vi "AirQualityViewer.vi"() -> ()   [LabVIEW 2020]
uses:
  Ctrls/StateMachineEnum.ctl
  Ctrls/ProgData.ctl
  user32.dll
panel:
  in  "Reload":bool
  in  "Settings":bool
  in  "Close":bool
  out "TitleBar":bool
  out "Data":timestamp format="%<%H:%M %d/%m/%y>T"
  out "Value":dbl
  out "Main Graph":cluster{timestamp[], dbl[]}[](graph)
  in  "Sensors":u16(ring) items=["dwutlenek azotu", "ozon"]
  # "Mierzony parametr:"
  # "Zaznaczony punkt:"
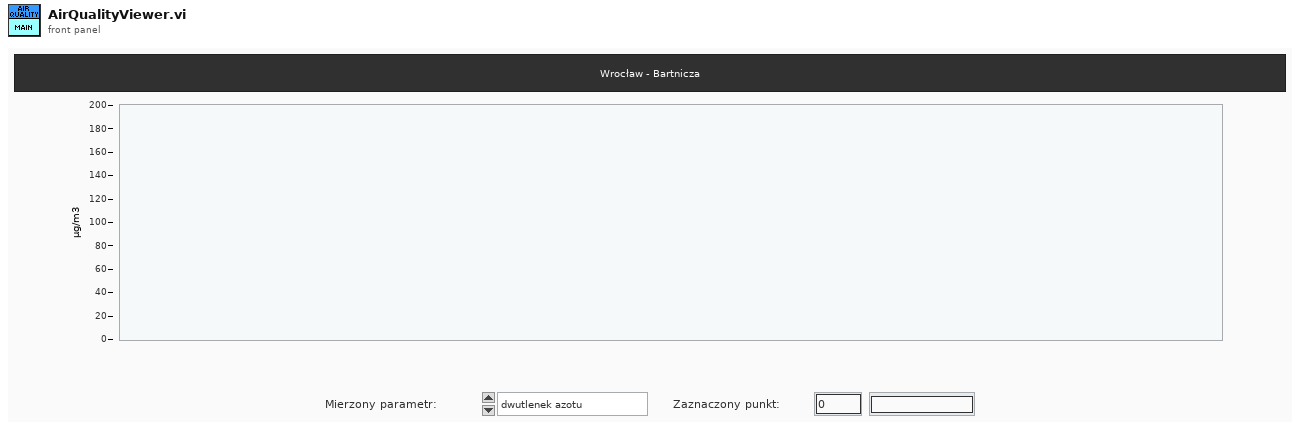
[diagram p1: front panel]
types:
  T1 = typedef "ProgData.ctl" = cluster{"Station":string[], "Sensor List":string[], "Sensor Id":dbl[], "Parameters":string[], "Values":i32[]}
  T2 = typedef "StateMachineEnum.ctl" = enum16{"INIT", "IDLE", "GET DATA", "ERROR HANDLER", "CLOSE"}
  T3 = typedef "LVPointDoubleTypeDef.ctl" = cluster{"Cursor X":dbl, "Cursor Y":dbl}
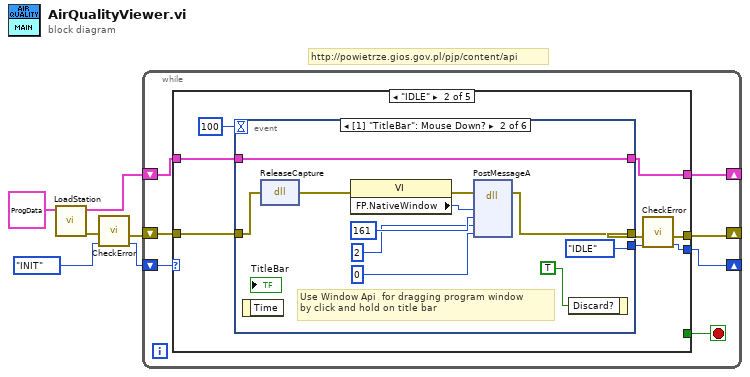
[diagram p0: block diagram]
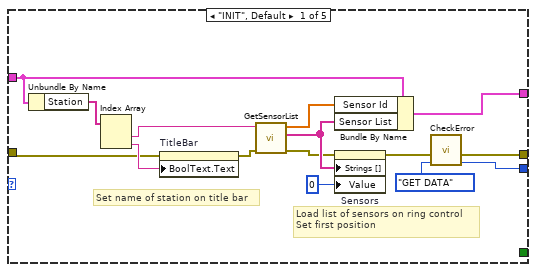
[diagram p2: hidden frame]
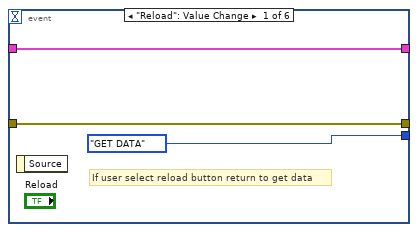
[diagram p3: hidden frame]
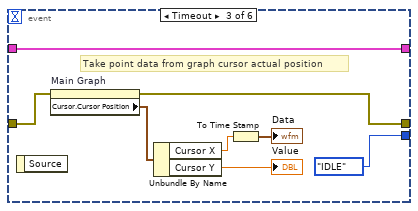
[diagram p4: hidden frame]
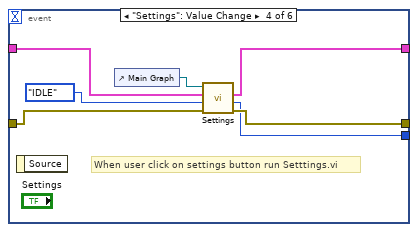
[diagram p5: hidden frame]
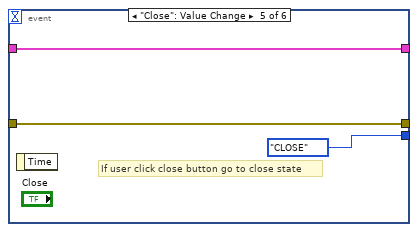
[diagram p6: hidden frame]
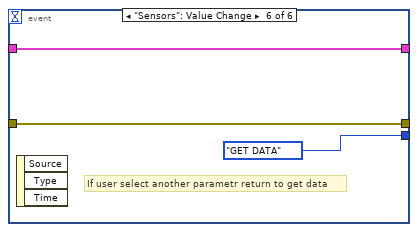
[diagram p7: hidden frame]
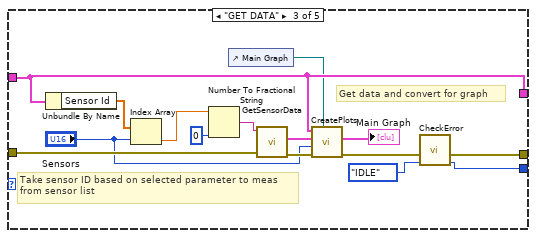
[diagram p8: hidden frame]
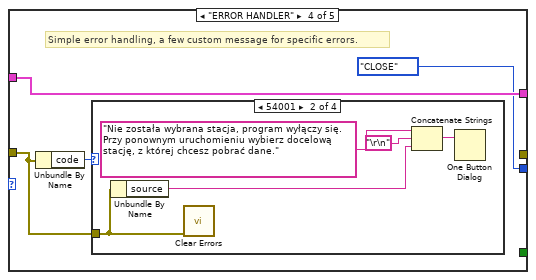
[diagram p9: hidden frame]
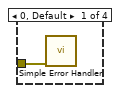
[diagram p10: hidden frame]
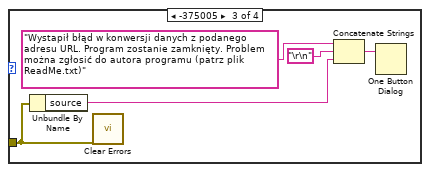
[diagram p11: hidden frame]
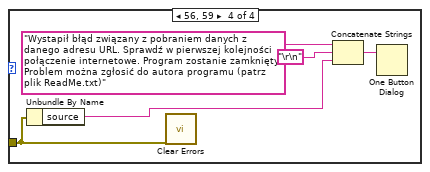
[diagram p12: hidden frame]
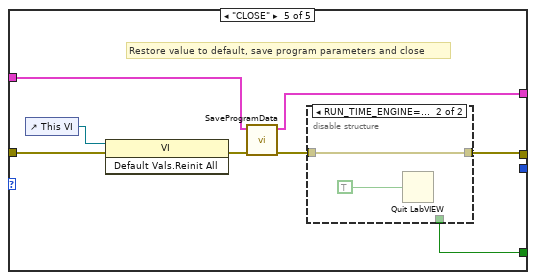
[diagram p13: hidden frame]
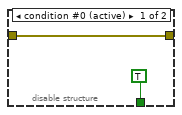
[diagram p14: hidden frame]
diagram:
  # "http://powietrze.gios.gov.pl/pjp/content/api"
  n1 = call "LoadStation.vi"("Prog Data In"=T1 {"Station"=[], "Sensor List"=[], "Sensor Id"=[], "Parameters"=["PM10", "PM2.5", "ozon", "dwutlenek azotu", "dwutlenek siarki", "benzen", "tlenek węgla"], "Values"=[110, 75, 180, 200, 350, 21, 15]}) -> ("Error Out"=w4:errorcluster, "Prog Data Out"=w5:T1)  [unwired: 9 in]
  n2 = call "CheckError.vi"("State In"=StateMachineEnum."INIT", "Error In"=w4) -> ("State Out"=w1:T2, "Error Out"=w3:errorcluster)  [unwired: 8 in]
  n3 = while {
    shift-right: [w8] -> _
    shift-left: w3 -> [w12]
    shift-right: [w9] -> _
    shift-left: w1 -> [w13]
    shift-right: [w10] -> _
    shift-left: w5 -> [w11]
    stop <- w7 stop-if-true
    n4 = case shown="\"IDLE\"" w13 {
      tunnel: w12 -> [w15 w36 w86 w88 w114]
      tunnel: w11 -> [w19 w31 w77 w90 w108]
      tunnel: [w28 w30 w77 w90 w107] -> w10
      tunnel: [w21 w35 w79 StateMachineEnum."CLOSE" ("State Out") _] -> w9
      tunnel: [w20 w34 w81 _ w112] -> w8
      tunnel: [_ _ _ _ w111] -> w7
      frame "INIT", Default {
        # "Load list of sensors on ring control\nSet first position"
        # "Set name of station on title bar"
        n5 = Unbundle By Name(w19) -> ("Station"=w18:string[])
        n6 = Index Array(array=w18) -> (element #1=w27:string, element #2=w16:string)  [unwired: 2 in]
        n7 = property on="TitleBar" class="Bool (strict)"(error in=w15, "BoolText.Text"=w16) -> (error out=w14:errorcluster)  [unwired: 1 in, 1 out]
        n8 = call "GetSensorList.vi"("Error In"=w14, "Station Id"=w27) -> ("Error Out"=w24:errorcluster, "Sensor List"=w25:string[], "Sensor Id"=w26:dbl[])  [unwired: 7 in]
        n9 = Bundle By Name(cluster=w19, "Sensor Id"=w26, "Sensor List"=w25) -> (w28:T1)
        n10 = property on="Sensors" class="Ring (strict)"(error in=w24, "Strings []"=w25, "Value"=0) -> (error out=w23:errorcluster)  [unwired: 1 in, 1 out]
        n11 = call "CheckError.vi"("State In"=StateMachineEnum."GET DATA", "Error In"=w23) -> ("State Out"=w21:T2, "Error Out"=w20:errorcluster)  [unwired: 8 in]
      }
      frame "IDLE" {
        n12 = event shown="[1] \"TitleBar\": Mouse Down?" {
          selector: _ -> [_ _ _ _ _ _]
          dyn-events: _ -> [_ _ _ _ _ _]
          timeout: 100 -> [_ _ _ _ _ _]
          tunnel: w36 -> [w38 w43 w58 w65 w67 w71]
          tunnel: [StateMachineEnum."GET DATA" ("State In") StateMachineEnum."IDLE" ("State In") StateMachineEnum."IDLE" ("State In") w59 StateMachineEnum."CLOSE" ("State In") StateMachineEnum."GET DATA" ("State In")] -> w33
          tunnel: [w38 w42 w57 w64 w67 w71] -> w32
          tunnel: w31 -> [w37 w40 w51 w62 w66 w70]
          tunnel: [w37 w40 w51 w61 w66 w70] -> w30
          event "Reload": Value Change {
            # "If user select reload button return to get data"
            n13 = event-data() -> ()  [unwired: 1 in, 1 out]
          }
          event "TitleBar": Mouse Down? {
            # "Use Window Api  for dragging program window\nby click and hold on title bar"
            n14 = event-data() -> ()  [unwired: 1 in, 1 out]
            n15 = dll-call lib="user32.dll" fn="ReleaseCapture"(error in=w43) -> (error out=w47:errorcluster)  [unwired: 3 in, 1 out]
            n16 = property class="VI"(error in=w47) -> (error out=w48:errorcluster, "FP.NativeWindow"=w49:u64)  [unwired: 1 in, 1 out]
            n17 = dll-call lib="user32.dll" fn="PostMessageA"(error in=w48, "hWnd"=w49, "Msg"=161, "wParam"=2, "lParam"=0) -> (error out=w42:errorcluster)  [unwired: 7 in, 1 out]
            n18 = event-data("Discard?"=TRUE) -> ()  [unwired: 1 in, 1 out]
          }
          event Timeout {
            # "Take point data from graph cursor actual position"
            n19 = event-data() -> ()  [unwired: 1 in, 1 out]
            n20 = property on="Main Graph" class="XYGraph (strict)"(error in=w58) -> (error out=w57:errorcluster, "Cursor.Cursor Position"=w56:T3)  [unwired: 1 in, 1 out]
            n21 = Unbundle By Name(w56) -> ("Cursor X"=w53:dbl, "Cursor Y"=→"Value":dbl)
            n22 = To Time Stamp(1:w53) -> (0:→"Data":timestamp)
          }
          event "Settings": Value Change {
            # "When user click on settings button run Setttings.vi"
            n23 = event-data() -> ()  [unwired: 1 in, 1 out]
            n24 = control-ref of="Main Graph"() -> (w60:refnum<vi>)
            n25 = call "Settings.vi"("Error In"=w65, "State In"=StateMachineEnum."IDLE", "Proga Data In"=w62, "Main Graph"=w60) -> ("Error Out"=w64:errorcluster, "State Out"=w59:T2, "Prog Data Out"=w61:T1)  [unwired: 5 in]
          }
          event "Close": Value Change {
            # "If user click close button go to close state"
            n26 = event-data() -> ()  [unwired: 1 in, 1 out]
          }
          event "Sensors": Value Change {
            # "If user select another parametr return to get data"
            n27 = event-data() -> ()  [unwired: 1 in, 3 out]
          }
        }
        n28 = call "CheckError.vi"("State In"=w33, "Error In"=w32) -> ("State Out"=w35:T2, "Error Out"=w34:errorcluster)  [unwired: 8 in]
      }
      frame "GET DATA" {
        # "Get data and convert for graph"
        # "Take sensor ID based on selected parameter to meas \nfrom sensor list"
        n29 = Unbundle By Name(w77) -> ("Sensor Id"=w85:dbl[])
        n30 = Index Array(array=w85, index="Sensors") -> (element=w82:dbl)
        n31 = Number To Fractional String(number=w82, precision (6)=i16 0) -> (F-format string=w83:string)  [unwired: 2 in]
        n32 = control-ref of="Main Graph"() -> (w72:refnum<vi>)
        n33 = call "GetSensorData.vi"("Error In"=w86, "Sensor id"=w83) -> ("Error Out"=w78:errorcluster, "Data Out"=w76:cluster{"Dates":timestamp[], "Values":dbl[]})  [unwired: 8 in]
        n34 = call "CreatePlots.vi"("Main Graph"=w72, "Error In"=w78, "Sensors"="Sensors", "Plot data In"=w76, "Prog data In"=w77) -> ("Error Out"=w74:errorcluster, "XY Plots"=→"Main Graph":cluster{"Dates":timestamp[], "Values":dbl[]}[])  [unwired: 5 in]
        n35 = call "CheckError.vi"("State In"=StateMachineEnum."IDLE", "Error In"=w74) -> ("State Out"=w79:T2, "Error Out"=w81:errorcluster)  [unwired: 8 in]
      }
      frame "ERROR HANDLER" {
        # "Simple error handling, a few custom message for specific errors."
        n36 = Unbundle By Name(w88) -> ("code"=w89:i32)
        n37 = case shown="54001" w89 {
          tunnel: w88 -> [w91 w95 w99 w104]
          frame 0, Default {
            n38 = call <vilib>:"Simple Error Handler.vi"("error in (no error)"=w91) -> ()  [unwired: 4 in, 5 out]
          }
          frame 54001 {
            n39 = Unbundle By Name(w95) -> ("source"=w94:string)
            n40 = call <vilib>:"Clear Errors.vi"("error in (no error)"=w95) -> ()  [unwired: 5 in, 2 out]
            n41 = Concatenate Strings("Nie została wybrana stacja, program wyłączy się. Przy ponownym uruchomieniu wybierz docelową stację, z której chcesz pobrać dane." ("message"), "\r\n", w94) -> (w92:string)
            n42 = One Button Dialog(message=w92) -> ()  [unwired: 1 in, 1 out]
          }
          frame -375005 {
            n43 = Unbundle By Name(w99) -> ("source"=w98:string)
            n44 = call <vilib>:"Clear Errors.vi"("error in (no error)"=w99) -> ()  [unwired: 5 in, 2 out]
            n45 = Concatenate Strings("Wystapił błąd w konwersji danych z podanego adresu URL. Program zostanie zamknięty. Problem można zgłosić do autora programu (patrz plik ReadMe.txt)" ("message"), "\r\n", w98) -> (w97:string)
            n46 = One Button Dialog(message=w97) -> ()  [unwired: 1 in, 1 out]
          }
          frame 56, 59 {
            n47 = Unbundle By Name(w104) -> ("source"=w103:string)
            n48 = call <vilib>:"Clear Errors.vi"("error in (no error)"=w104) -> ()  [unwired: 5 in, 2 out]
            n49 = Concatenate Strings("Wystapił błąd związany z pobraniem danych z danego adresu URL. Sprawdź w pierwszej kolejności połączenie internetowe. Program zostanie zamknięty. Problem można zgłosić do autora programu (patrz plik ReadMe.txt)" ("message"), "\r\n", w103) -> (w105:string)
            n50 = One Button Dialog(message=w105) -> ()  [unwired: 1 in, 1 out]
          }
        }
      }
      frame "CLOSE" {
        # "Restore value to default, save program parameters and close"
        n51 = control-ref of="This VI"() -> (w113:refnum<vi>)
        n52 = invoke class="VI" method="Default Vals.Reinit All"(reference=w113, error in=w114) -> (error out=w110:errorcluster)  [unwired: 1 in, 2 out]
        n53 = call "SaveProgramData.vi"("Error In"=w110, "Prog Data In"=w108) -> ("Error Out"=w109:errorcluster, "Prog Data Out"=w107:T1)  [unwired: 8 in]
        n54 = disable-structure shown="RUN_TIME_ENGINE==True" {
          disable-tunnel: w109 -> [w116 w117]
          disable-tunnel: [w116 w117] -> w112
          disable-tunnel: [TRUE _] -> w111
          frame condition #0 (active) {
          }
          frame condition #1 {
            n55 = Quit LabVIEW(quit? (T)=TRUE) -> ()
          }
        }
      }
    }
  }
